vi "Barcode-Indentify-Sort(Include-Read)_Api.vi"(8 "Error In":errorcluster, 11 "Progressing Data":T5) -> (0 "Error Out":errorcluster, 1 "輸出顏色-位置":T1(array[cluster]), 2 "Image":T2(plugin-control), 3 "Progressing Data":T5, 4 "第一次輸出結果(含排序)":cluster{"X值":dbl, "Data":string}[](array[cluster]), 5 "Barcodes":T3(array[cluster]) {"Confidence Level" format="%.2f"; "Barcode Type" items=["Reserved", "Codabar", "Code 39", "Code 93", "Code 128", "EAN 8", "EAN 13", "Interleaved 2 of 5", "MSI", "UPCA", "Pharmacode", "RSS Limited"]; "Bounding Box"."y" format="%.2f"; "Bounding Box"."x" format="%.2f"})   [LabVIEW 2019]
uses:
  <vilib>/vision/Image Controls.llb/IMAQ Image.ctl
  <vilib>/userDefined/High Color/IMAQdx.ctl
  <vilib>/myRIO/Instrument Drivers/Onboard IO/DIO/typedefs/DIO Reference.ctl
  <vilib>/myRIO/Common/Instrument Driver Framework/Utilities/typedefs/myRIO Generic Hardware Reference.ctl
  <vilib>/myRIO/Common/Instrument Driver Framework/Utilities/typedefs/Hardware Version Enum.ctl
  <vilib>/myRIO/Common/Instrument Driver Framework/Utilities/typedefs/myRIO v1.0 Reference.ctl
  <vilib>/myRIO/Common/Instrument Driver Framework/Utilities/typedefs/Generic FPGA Reference.ctl
  <vilib>/myRIO/Common/Instrument Driver Framework/myRIO v1.0/DIO/typedefs/DIO Channels List.ctl
  <vilib>/myRIO/Common/Instrument Driver Framework/myRIO v1.0/DIO/typedefs/DIO Channels Enum.ctl
  <vilib>/userDefined/High Color/nirio_resource_hc.ctl
  <vilib>/myRIO/Common/Instrument Driver Framework/Utilities/vis/Is FPGA Ref Available.vi
  <vilib>/myRIO/Common/Instrument Driver Framework/myRIO v1.0/DIO/vis/myRIO v1.1 Open DIO.vi
  <vilib>/myRIO/Instrument Drivers/Onboard IO/DIO/vis/Write.vi
  <vilib>/myRIO/Common/Instrument Driver Framework/Utilities/vis/Validate Channels.vi
  <vilib>/myRIO/Common/Instrument Driver Framework/myRIO v1.0/DIO/vis/myRIO v1.0 Reserve DIO.vi
  <vilib>/myRIO/Common/Instrument Driver Framework/myRIO v1.0/Resource Manager/vis/myRIO v1.0 Reserve Channel List.vi
  <vilib>/myRIO/Common/Instrument Driver Framework/myRIO v1.0/DIO/vis/myRIO v1.0 Build MUX Configuration DIO.vi
  <vilib>/myRIO/Common/Instrument Driver Framework/myRIO v1.0/Resource Manager/vis/myRIO v1.0 Reserve Channel.vi
  <vilib>/myRIO/Common/Instrument Driver Framework/myRIO v1.0/Resource Manager/vis/myRIO v1.0 Unreserve Channel.vi
  <vilib>/myRIO/Common/Instrument Driver Framework/myRIO v1.0/Resource Manager/vis/myRIO v1.0 Create Configuration List.vi
  <vilib>/myRIO/Common/Instrument Driver Framework/myRIO v1.0/Resource Manager/vis/myRIO v1.0 Build Mutex Name.vi
  <vilib>/Utility/VariantDataType/GetNumericInfo.vi
  <vilib>/Utility/error.llb/Error Cluster From Error Code.vi
  <vilib>/myRIO/Common/Instrument Driver Framework/myRIO v1.0/myRIO v1.1 Open.vi
  <vilib>/myRIO/Common/Instrument Driver Framework/Utilities/vis/IO Manager.vi
  <vilib>/myRIO/Common/Instrument Driver Framework/Utilities/vis/Configuration Manager.vi
  <vilib>/myRIO/Common/Instrument Driver Framework/myRIO v1.0/Resource Manager/vis/myRIO v1.0 Configure IO.vi
  <vilib>/myRIO/Common/Instrument Driver Framework/myRIO v1.0/myRIO v1.0 Close.vi
  <vilib>/myRIO/Common/Instrument Driver Framework/myRIO v1.0/DIO/vis/myRIO v1.0 Write DIO.vi
  <vilib>/myRIO/Express VI/Onboard Devices/LED/LED Express VI.xnode
  <vilib>/myRIO/Instrument Drivers/Onboard IO/DIO/vis/myRIO DIO Open.xnode
  <vilib>/myRIO/Instrument Drivers/Onboard IO/DIO/DIO.lvlib
panel:
  out "第二次輸出結果(含排序)":cluster{"x":dbl, "Data":string}[](array[cluster])
  out "排完順序的辨識結果":cluster{"Numeric":dbl, "Data":string}[](array[cluster])
  in  "Stop 2":bool
  out "Image 2":T2(plugin-control)
  out "Barcodes 2":T3(array[cluster]) {"Confidence Level" format="%.2f"; "Barcode Type" items=["Reserved", "Codabar", "Code 39", "Code 93", "Code 128", "EAN 8", "EAN 13", "Interleaved 2 of 5", "MSI", "UPCA", "Pharmacode", "RSS Limited"]; "Bounding Box"."y" format="%.2f"; "Bounding Box"."x" format="%.2f"}
  in  "Stop":bool
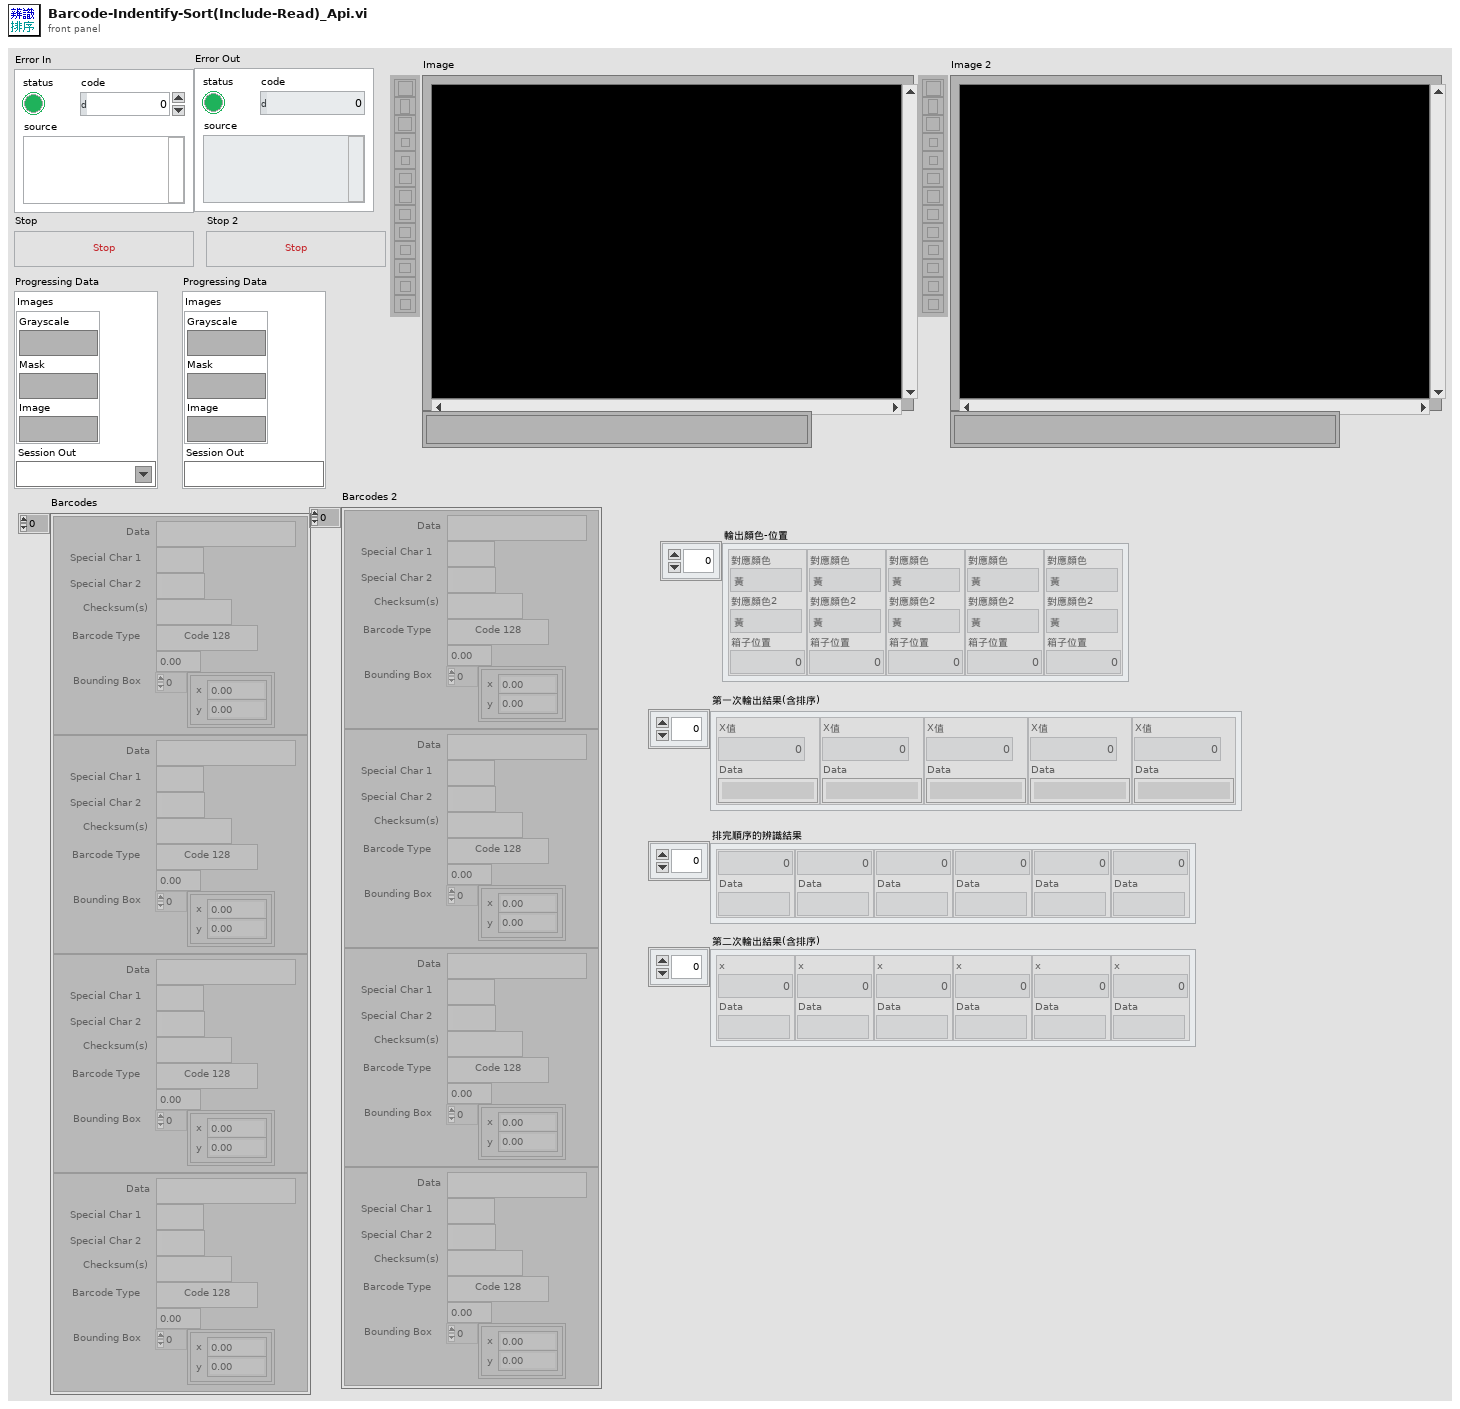
[diagram p1: front panel]
types:
  T1 = cluster{"對應顏色":enum16{"黃", "紅", "綠", "藍", "黑"}, "對應顏色2":enum16{"黃", "紅", "綠", "藍", "黑"}, "箱子位置":i32}[]
  T2 = typedef "IMAQ Image.ctl" = refnum<image>
  T3 = cluster{"Data":string, "Special Char 1":string, "Special Char 2":string, "Checksum(s)":string, "Barcode Type":u32, "Confidence Level":sgl, "Bounding Box":cluster{"x":sgl, "y":sgl}[]}[]
  T4 = typedef "IMAQdx.ctl" = refnum<k21>
  T5 = cluster{"Images":cluster{"Grayscale":T2, "Mask":T2, "Image":T2}, "Session Out":T4}
  T6 = typedef "DIO.lvlib/DIO Reference.ctl" = cluster{"myRIO Reference":T7, "DIO Channels List":T11}
  T7 = typedef "myRIO Generic Hardware Reference.ctl" = cluster{"myRIO Model":T8, "myRIO Hardware Reference":T9}
  T8 = typedef "Hardware Version Enum.ctl" = enum16{"Unknown", "myRIO-1900", "myRIO-1950", "roboRIO", "NI ELVIS RIO CM", "ELVIS III"}
  T9 = typedef "myRIO v1.0 Reference.ctl" = cluster{"Generic FPGA Reference":T10, "Allow multiple opens":bool}
  T10 = typedef "Generic FPGA Reference.ctl" = refnum<k20>
  T11 = typedef "DIO Channels List.ctl" = T12[]
  T12 = typedef "DIO Channels Enum.ctl" = enum16{"Not Connected", "C/DIO0", "C/DIO1", "C/DIO2", "C/DIO3", "C/DIO4", "C/DIO5", "C/DIO6", "C/DIO7", "A/DIO0", "A/DIO1", "A/DIO2", "A/DIO3", "A/DIO4", "A/DIO5", "A/DIO6", "A/DIO7", "A/DIO8", "A/DIO9", "A/DIO10", "A/DIO11", "A/DIO12", "A/DIO13", "A/DIO14", "A/DIO15", "A/DIO16", "A/DIO17", "A/DIO18", "A/DIO19", "B/DIO0", "B/DIO1", "B/DIO2", "B/DIO3", "B/DIO4", "B/DIO5", "B/DIO6", "B/DIO7", "B/DIO8", "B/DIO9", "B/DIO10", "B/DIO11", "B/DIO12", "B/DIO13", "B/DIO14", "B/DIO15", "B/DIO16", "B/DIO17", "B/DIO18", "B/DIO19", "LED0", "LED1", "LED2", "LED3", "Button0", "DIO/DIO0", "DIO/DIO1", "DIO/DIO2", "DIO/DIO3", "DIO/DIO4", "DIO/DIO5", "DIO/DIO6", "DIO/DIO7", "DIO/DIO8", "DIO/DIO9", "SPI/CS0", "SPI/CS1", "SPI/CS2", "SPI/CS3", "LED RADIO (Green)", "LED RADIO (Red)", "LED COMM (Green)", "LED COMM (Red)", "LED MODE (Green)", "LED MODE (Red)"}
  T13 = typedef "nirio_resource_hc.ctl" = tag
  T14 = cluster{"對應顏色":enum16{"黃", "紅", "綠", "藍", "黑"}, "對應顏色2":enum16{"黃", "紅", "綠", "藍", "黑"}, "箱子位置":i32}
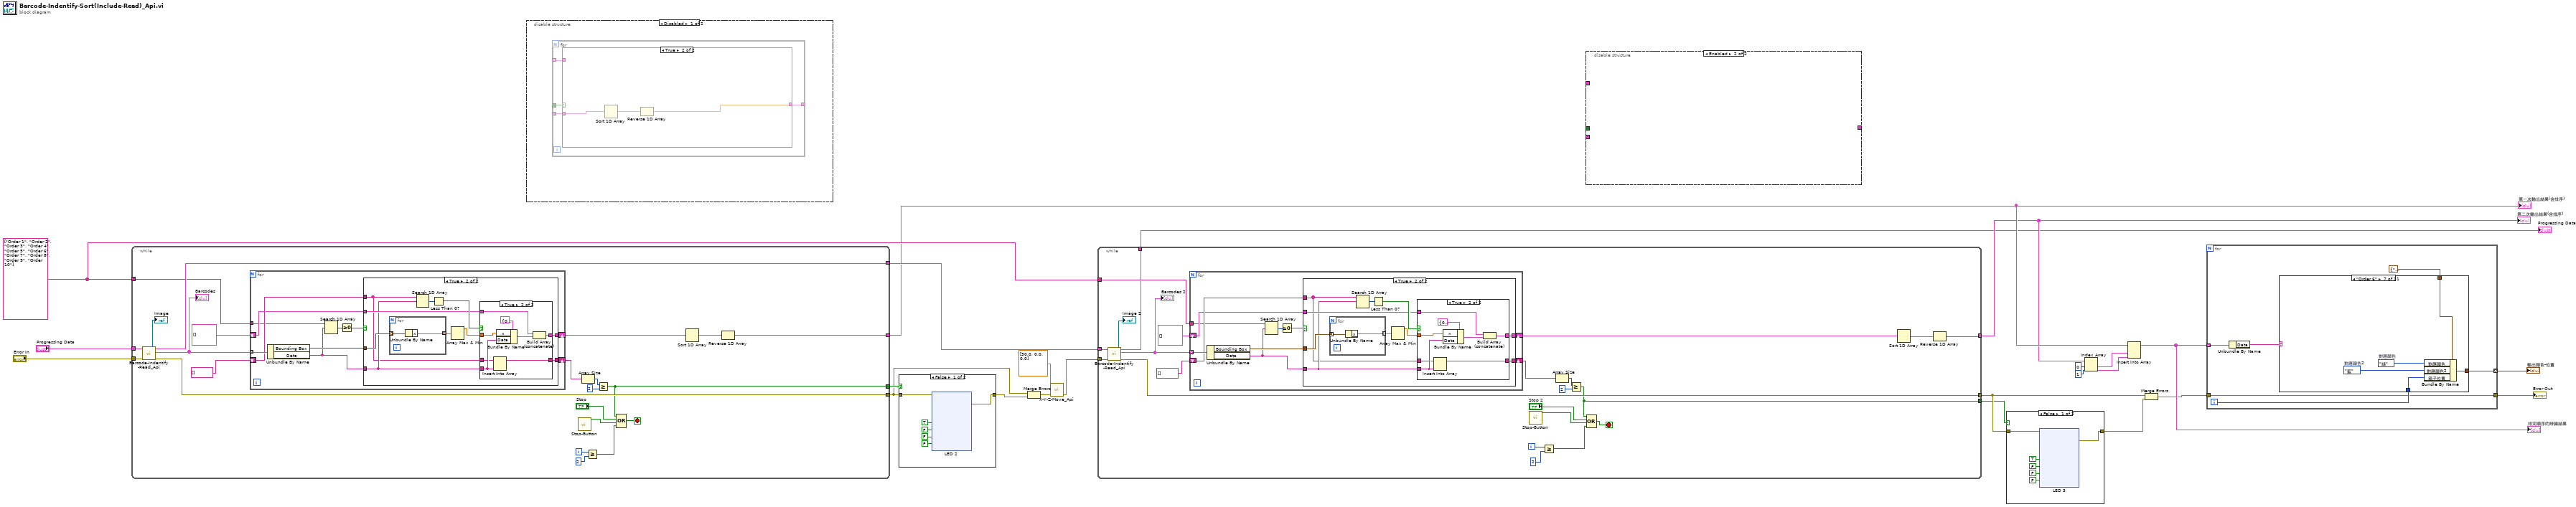
[diagram p0: block diagram]
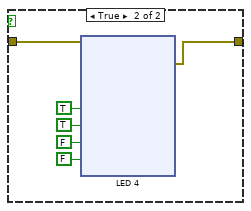
[diagram p2: hidden frame]
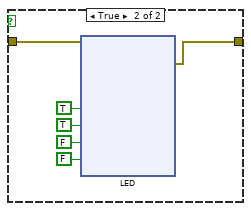
[diagram p3: hidden frame]
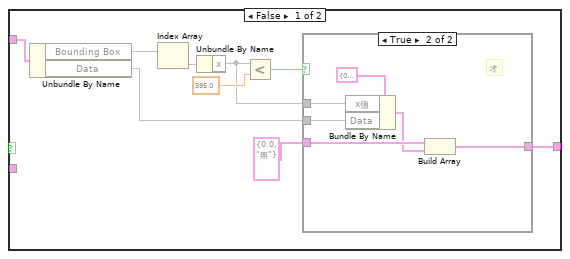
[diagram p4: hidden frame]
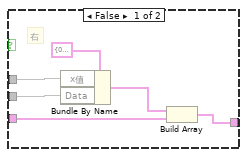
[diagram p5: hidden frame]
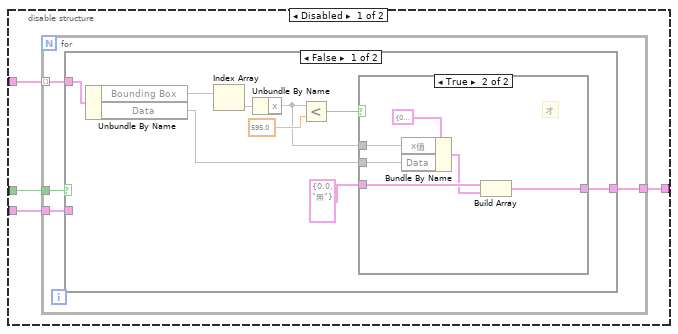
[diagram p7: hidden frame]
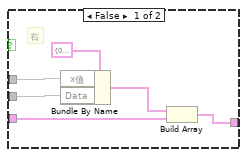
[diagram p8: hidden frame]
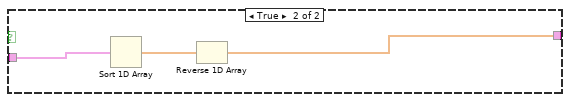
[diagram p9: hidden frame]
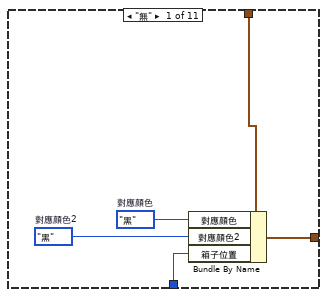
[diagram p10: hidden frame]
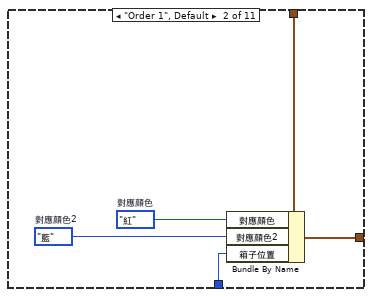
[diagram p11: hidden frame]
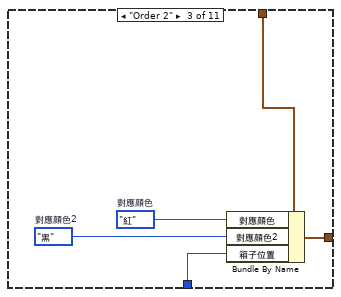
[diagram p12: hidden frame]
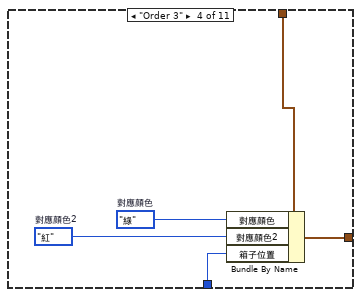
[diagram p13: hidden frame]
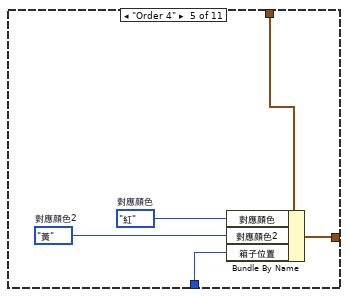
[diagram p14: hidden frame]
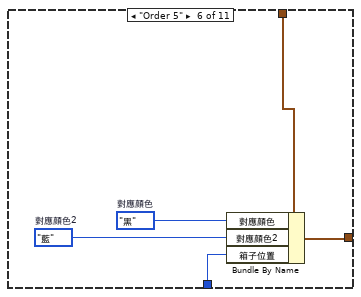
[diagram p15: hidden frame]
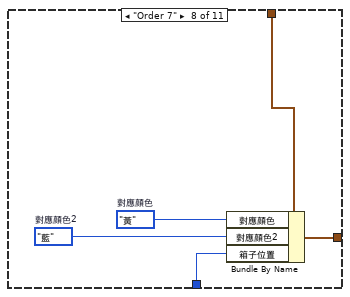
[diagram p16: hidden frame]
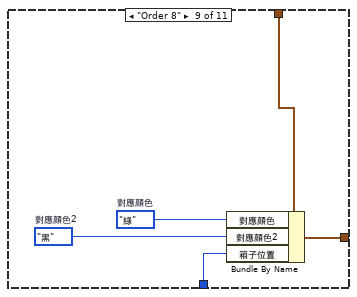
[diagram p17: hidden frame]
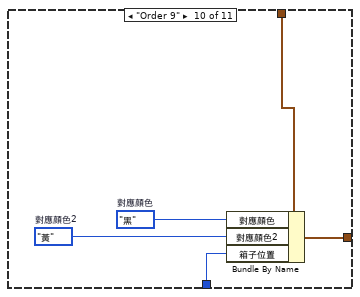
[diagram p18: hidden frame]
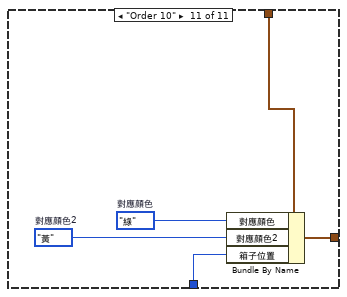
[diagram p19: hidden frame]
diagram:
  w21 = string[] ["Order 1", "Order 2", "Order 3", "Order 4", "Order 5", "Order 6", "Order 7", "Order 8", "Order 9", "Order 10"]
  n1 = while {
    tunnel: "Error In" -> [w33]
    tunnel: [w26] -> w14
    tunnel: [w34] -> w5
    tunnel: "Progressing Data" -> [w40]
    tunnel: [w39] -> w22
    tunnel: w21 -> [w36]
    tunnel: [w25] -> w8
    i -> [w32]
    stop <- w42 stop-if-true
    n2 = call "Barcode-Indentify-Read_Api.vi"("Error In"=w33, "Progressing Data"=w40) -> ("Error Out"=w34:errorcluster, "Barcodes"=w29:T3, "Progressing Data"=w39:T5, "Image"=→"Image":T2)  [unwired: 6 in]
    "Barcodes" <- w29
    n3 = for {
      tunnel: w29 -> [w56] mode=indexing
      shift-right: [w51] -> w35
      shift-left: string[] [] -> [w53]
      shift-right: [w54] -> w27
      shift-left: cluster{sgl, "Data":string}[] [] -> [w52]
      tunnel: w36 -> [w48]
      n4 = Unbundle By Name(w56) -> ("Bounding Box"=w55:cluster{"x":sgl, "y":sgl}[], "Data"=w47:string)
      n5 = Search 1D Array(1D array=w48, element=w47) -> (index of element=w50:i32)  [unwired: 1 in]
      n6 = Greater Or Equal To 0?(x=w50) -> (x >= 0?=w49:bool)
      n7 = case shown="True" w49 {
        tunnel: w55 -> [_ w68]
        tunnel: [w57 w66] -> w54
        tunnel: w47 -> [_ w61]
        tunnel: w53 -> [w58 w60]
        tunnel: w52 -> [w57 w63]
        tunnel: [w58 w62] -> w51
        frame False {
        }
        frame True {
          n8 = for {
            tunnel: w68 -> [w80] mode=indexing
            tunnel: [w79] -> w67 mode=indexing
            n9 = Unbundle By Name(w80) -> ("x"=w79:sgl)
          }
          n10 = Search 1D Array(1D array=w60, element=w61) -> (index of element=w65:i32)  [unwired: 1 in]
          n11 = Less Than 0?(x=w65) -> (x < 0?=w64:bool)
          n12 = Array Max & Min(array=w67) -> (max value=w59:sgl)  [unwired: 3 out]
          n13 = case shown="True" w64 {
            tunnel: w59 -> [_ w78]
            tunnel: w61 -> [_ w76]
            tunnel: [w69 w77] -> w66
            tunnel: w60 -> [w70 w75]
            tunnel: [w70 w74] -> w62
            tunnel: w63 -> [w69 w73]
            frame False {
            }
            frame True {
              n14 = Insert Into Array "Insert Into Array"(array=w75, new element=w76) -> (w74:string[])  [unwired: 1 in]
              n15 = Bundle By Name(cluster=cluster{"x":dbl, "Data":string} {"x"=0.0, "Data"=""} ("input cluster"), "x"=w78, "Data"=w76) -> (w72:cluster{"x":dbl, "Data":string})
              n16 = Build Array (concatenate)(w73, w72) -> (w77:cluster{"x":dbl, "Data":string}[])
            }
          }
        }
      }
    }
    n17 = call "Stop-Button.vi"() -> ("顯示按下?"=w38:bool)  [unwired: 10 in, 1 out]
    n18 = Array Size(array=w35) -> (size(s)=w44:i32)
    n19 = Greater Or Equal?(x=w32, y=2) -> (x >= y?=w31:bool)
    n20 = Greater Or Equal?(x=w44, y=2) -> (x >= y?=w25:bool)
    n21 = Compound Arithmetic op=OR(w25, "Stop", w38, w31) -> (w42:bool)
    n22 = Sort 1D Array(array=w27) -> (sorted array=w28:cluster{"x":dbl, "Data":string}[])
    n23 = Reverse 1D Array(array=w28) -> (reversed array=w26:cluster{"x":dbl, "Data":string}[])
  }
  "第一次輸出結果(含排序)" <- w14
  n24 = disable-structure shown="Disabled" {
    frame Disabled {
      n25 = for {
        tunnel: [w84] -> _
        tunnel: _ -> [w83]
        tunnel: _ -> [w82]
        tunnel: _ -> [w81] mode=indexing
        n26 = case shown="True" w82 {
          tunnel: [w85 w108] -> w84
          tunnel: w83 -> [_ w106]
          tunnel: w81 -> [w89 _]
          frame False {
            n27 = Unbundle By Name(w89) -> ("Bounding Box"=w93, "Data"=w88)
            n28 = Index Array(array=w93) -> (element=w92)  [unwired: 1 in]
            n29 = Unbundle By Name(w92) -> ("x"=w87)
            n30 = Less?(x=w87, y=sgl 595.0) -> (x < y?=w90:bool)
            n31 = case shown="True" w90 {
              tunnel: w88 -> [w98 w105]
              tunnel: w87 -> [w97 w104]
              tunnel: cluster{"x值":dbl, "Data":string} {"x值"=0.0, "Data"="無"} ("element") -> [w95 w101]
              tunnel: [w96 w102] -> w85
              frame False {
                # "右"
                n32 = Bundle By Name(cluster=cluster{"x值":dbl, "Data":string} {"x值"=0.0, "Data"=""} ("input cluster"), "x值"=w97, "Data"=w98) -> (w94:cluster{"x值":dbl, "Data":string})
                n33 = Build Array(w94, w95) -> (w96:cluster{"x值":dbl, "Data":string}[])
              }
              frame True {
                # "オ"
                n34 = Bundle By Name(cluster=cluster{"x值":dbl, "Data":string} {"x值"=0.0, "Data"=""} ("input cluster"), "x值"=w104, "Data"=w105) -> (w100:cluster{"x值":dbl, "Data":string})
                n35 = Build Array(w101, w100) -> (w102:cluster{"x值":dbl, "Data":string}[])
              }
            }
          }
          frame True {
            n36 = Sort 1D Array(array=w106) -> (sorted array=w107:ext[])
            n37 = Reverse 1D Array(array=w107) -> (reversed array=w108:ext[])
          }
        }
      }
    }
    frame Enabled {
    }
  }
  n38 = case shown="False" w8 {
    tunnel: w5 -> [w109 w158]
    tunnel: [w110 w153] -> w6
    frame False {
      n39 = xnode "LED 2"("LED0"=TRUE, "LED1"=FALSE, "LED2"=FALSE, "LED3"=FALSE, "error in (no error)"=w109) -> ("error out"=w110:errorcluster)
    }
    frame True {
      n40 = xnode "LED"("LED0"=TRUE, "LED1"=TRUE, "LED2"=FALSE, "LED3"=FALSE, "error in (no error)"=w158) -> ("error out"=w153:errorcluster)
    }
  }
  n41 = Merge Errors(w5, w6) -> (w7:errorcluster)
  n42 = call "X-Y-Z-Move_Api.vi"("Error In"=w7, "X-Y-Z移動"=dbl[] [50.0, 0.0, 0.0]) -> ("Error Out"=w23:errorcluster)  [unwired: 8 in, 1 out]
  n43 = while {
    tunnel: w23 -> [w217]
    tunnel: [w199] -> w13
    tunnel: [w206] -> w3
    tunnel: w22 -> [w211]
    tunnel: w21 -> [w208]
    tunnel: [w201] -> w9
    tunnel: [w197] -> w1
    i -> [w204]
    stop <- w213 stop-if-true
    n44 = call "Barcode-Indentify-Read_Api.vi"("Error In"=w217, "Progressing Data"=w211) -> ("Error Out"=w206:errorcluster, "Barcodes"=w202:T3, "Progressing Data"=w201:T5, "Image"=→"Image 2":T2)  [unwired: 6 in]
    "Barcodes 2" <- w202
    n45 = for {
      tunnel: w202 -> [w228] mode=indexing
      shift-right: [w223] -> w207
      shift-left: string[] [] -> [w225]
      shift-right: [w226] -> w198
      shift-left: cluster{sgl, "Data":string}[] [] -> [w224]
      tunnel: w208 -> [w220]
      n46 = Unbundle By Name(w228) -> ("Bounding Box"=w227:cluster{"x":sgl, "y":sgl}[], "Data"=w219:string)
      n47 = Search 1D Array(1D array=w220, element=w219) -> (index of element=w222:i32)  [unwired: 1 in]
      n48 = Greater Or Equal To 0?(x=w222) -> (x >= 0?=w221:bool)
      n49 = case shown="True" w221 {
        tunnel: w227 -> [_ w240]
        tunnel: [w229 w238] -> w226
        tunnel: w219 -> [_ w233]
        tunnel: w225 -> [w230 w232]
        tunnel: w224 -> [w229 w235]
        tunnel: [w230 w234] -> w223
        frame False {
        }
        frame True {
          n50 = for {
            tunnel: w240 -> [w252] mode=indexing
            tunnel: [w251] -> w239 mode=indexing
            n51 = Unbundle By Name(w252) -> ("x"=w251:sgl)
          }
          n52 = Search 1D Array(1D array=w232, element=w233) -> (index of element=w237:i32)  [unwired: 1 in]
          n53 = Less Than 0?(x=w237) -> (x < 0?=w236:bool)
          n54 = Array Max & Min(array=w239) -> (max value=w231:sgl)  [unwired: 3 out]
          n55 = case shown="True" w236 {
            tunnel: w231 -> [_ w250]
            tunnel: w233 -> [_ w248]
            tunnel: [w241 w249] -> w238
            tunnel: w232 -> [w242 w247]
            tunnel: [w242 w246] -> w234
            tunnel: w235 -> [w241 w245]
            frame False {
            }
            frame True {
              n56 = Insert Into Array "Insert Into Array"(array=w247, new element=w248) -> (w246:string[])  [unwired: 1 in]
              n57 = Bundle By Name(cluster=cluster{"x":dbl, "Data":string} {"x"=0.0, "Data"=""} ("input cluster"), "x"=w250, "Data"=w248) -> (w244:cluster{"x":dbl, "Data":string})
              n58 = Build Array (concatenate)(w245, w244) -> (w249:cluster{"x":dbl, "Data":string}[])
            }
          }
        }
      }
    }
    n59 = call "Stop-Button.vi"() -> ("顯示按下?"=w210:bool)  [unwired: 10 in, 1 out]
    n60 = Greater Or Equal?(x=w204, y=2) -> (x >= y?=w205:bool)
    n61 = Array Size(array=w207) -> (size(s)=w215:i32)
    n62 = Greater Or Equal?(x=w215, y=2) -> (x >= y?=w197:bool)
    n63 = Compound Arithmetic op=OR(w197, "Stop 2", w210, w205) -> (w213:bool)
    n64 = Sort 1D Array(array=w198) -> (sorted array=w200:cluster{"x":dbl, "Data":string}[])
    n65 = Reverse 1D Array(array=w200) -> (reversed array=w199:cluster{"x":dbl, "Data":string}[])
  }
  "Progressing Data" <- w9
  "第二次輸出結果(含排序)" <- w13
  n66 = disable-structure shown="Enabled" {
    disable-tunnel: _ -> [w256 _]
    disable-tunnel: _ -> [w255 _]
    disable-tunnel: _ -> [w254 _]
    disable-tunnel: [w253 _] -> _
    frame Disabled {
      n67 = for {
        tunnel: [w260] -> w253
        tunnel: w255 -> [w259]
        tunnel: w256 -> [w258]
        tunnel: w254 -> [w257] mode=indexing
        n68 = case shown="False" w258 {
          tunnel: [w261 w284] -> w260
          tunnel: w259 -> [_ w282]
          tunnel: w257 -> [w265 _]
          frame False {
            n69 = Unbundle By Name(w265) -> ("Bounding Box"=w269, "Data"=w264)
            n70 = Index Array(array=w269) -> (element=w268)  [unwired: 1 in]
            n71 = Unbundle By Name(w268) -> ("x"=w263)
            n72 = Less?(x=w263, y=sgl 595.0) -> (x < y?=w266:bool)
            n73 = case shown="True" w266 {
              tunnel: w264 -> [w274 w281]
              tunnel: w263 -> [w273 w280]
              tunnel: cluster{"x值":dbl, "Data":string} {"x值"=0.0, "Data"="無"} ("element") -> [w271 w277]
              tunnel: [w272 w278] -> w261
              frame False {
                # "右"
                n74 = Bundle By Name(cluster=cluster{"x值":dbl, "Data":string} {"x值"=0.0, "Data"=""} ("input cluster"), "x值"=w273, "Data"=w274) -> (w270:cluster{"x值":dbl, "Data":string})
                n75 = Build Array(w270, w271) -> (w272:cluster{"x值":dbl, "Data":string}[])
              }
              frame True {
                # "オ"
                n76 = Bundle By Name(cluster=cluster{"x值":dbl, "Data":string} {"x值"=0.0, "Data"=""} ("input cluster"), "x值"=w280, "Data"=w281) -> (w276:cluster{"x值":dbl, "Data":string})
                n77 = Build Array(w277, w276) -> (w278:cluster{"x值":dbl, "Data":string}[])
              }
            }
          }
          frame True {
            n78 = Sort 1D Array(array=w282) -> (sorted array=w283:ext[])
            n79 = Reverse 1D Array(array=w283) -> (reversed array=w284:ext[])
          }
        }
      }
    }
    frame Enabled {
    }
  }
  n80 = case shown="False" w1 {
    tunnel: w3 -> [w285 w334]
    tunnel: [w286 w329] -> w2
    frame False {
      n81 = xnode "LED 3"("LED0"=TRUE, "LED1"=FALSE, "LED2"=FALSE, "LED3"=FALSE, "error in (no error)"=w285) -> ("error out"=w286:errorcluster)
    }
    frame True {
      n82 = xnode "LED 4"("LED0"=TRUE, "LED1"=TRUE, "LED2"=FALSE, "LED3"=FALSE, "error in (no error)"=w334) -> ("error out"=w329:errorcluster)
    }
  }
  n83 = Index Array(array=w13, index #1=0 ("index"), index #2=1 ("index")) -> (element #1=w16:cluster{"x":dbl, "Data":string}, element #2=w15:cluster{"x":dbl, "Data":string})
  n84 = Insert Into Array(array=w14, new element #1=w16, new element #2=w15) -> (w12:cluster{"x":dbl, "Data":string}[])  [unwired: 1 in]
  "排完順序的辨識結果" <- w12
  n85 = Merge Errors(w3, w2) -> (w4:errorcluster)
  n86 = for {
    tunnel: [w377] -> w11 mode=indexing
    tunnel: w12 -> [w376] mode=indexing
    tunnel: [w374] -> w10
    tunnel: w4 -> [w374]
    i -> [w378]
    n87 = Unbundle By Name(w376) -> ("Data"=w375:string)
    n88 = case shown="\"Order 6\"" w375 {
      tunnel: w378 -> [w382 w388 w390 w396 w400 w405 w410 w415 w420 w425 w430]
      tunnel: [w383 w387 w391 w395 w401 w406 w411 w416 w421 w426 w431] -> w377
      tunnel: T14 {"對應顏色"=enum."黃", "對應顏色2"=enum."黃", "箱子位置"=0} ("input cluster") -> [w381 w384 w389 w394 w399 w404 w409 w414 w419 w424 w429]
      frame "無" {
        w379 = enum16{"黃", "紅", "綠", "藍", "黑"}."黑"  # 對應顏色2
        w380 = enum16{"黃", "紅", "綠", "藍", "黑"}."黑"  # 對應顏色
        n89 = Bundle By Name(cluster=w381, "對應顏色"=w380, "對應顏色2"=w379, "箱子位置"=w382) -> (w383:T14)
      }
      frame "Order 1", Default {
        w385 = enum16{"黃", "紅", "綠", "藍", "黑"}."藍"  # 對應顏色2
        w386 = enum16{"黃", "紅", "綠", "藍", "黑"}."紅"  # 對應顏色
        n90 = Bundle By Name(cluster=w384, "對應顏色"=w386, "對應顏色2"=w385, "箱子位置"=w388) -> (w387:T14)
      }
      frame "Order 2" {
        w392 = enum16{"黃", "紅", "綠", "藍", "黑"}."黑"  # 對應顏色2
        w393 = enum16{"黃", "紅", "綠", "藍", "黑"}."紅"  # 對應顏色
        n91 = Bundle By Name(cluster=w389, "對應顏色"=w393, "對應顏色2"=w392, "箱子位置"=w390) -> (w391:T14)
      }
      frame "Order 3" {
        w397 = enum16{"黃", "紅", "綠", "藍", "黑"}."紅"  # 對應顏色2
        w398 = enum16{"黃", "紅", "綠", "藍", "黑"}."綠"  # 對應顏色
        n92 = Bundle By Name(cluster=w394, "對應顏色"=w398, "對應顏色2"=w397, "箱子位置"=w396) -> (w395:T14)
      }
      frame "Order 4" {
        w402 = enum16{"黃", "紅", "綠", "藍", "黑"}."黃"  # 對應顏色2
        w403 = enum16{"黃", "紅", "綠", "藍", "黑"}."紅"  # 對應顏色
        n93 = Bundle By Name(cluster=w399, "對應顏色"=w403, "對應顏色2"=w402, "箱子位置"=w400) -> (w401:T14)
      }
      frame "Order 5" {
        w407 = enum16{"黃", "紅", "綠", "藍", "黑"}."藍"  # 對應顏色2
        w408 = enum16{"黃", "紅", "綠", "藍", "黑"}."黑"  # 對應顏色
        n94 = Bundle By Name(cluster=w404, "對應顏色"=w408, "對應顏色2"=w407, "箱子位置"=w405) -> (w406:T14)
      }
      frame "Order 6" {
        w412 = enum16{"黃", "紅", "綠", "藍", "黑"}."藍"  # 對應顏色2
        w413 = enum16{"黃", "紅", "綠", "藍", "黑"}."綠"  # 對應顏色
        n95 = Bundle By Name(cluster=w409, "對應顏色"=w413, "對應顏色2"=w412, "箱子位置"=w410) -> (w411:T14)
      }
      frame "Order 7" {
        w417 = enum16{"黃", "紅", "綠", "藍", "黑"}."藍"  # 對應顏色2
        w418 = enum16{"黃", "紅", "綠", "藍", "黑"}."黃"  # 對應顏色
        n96 = Bundle By Name(cluster=w414, "對應顏色"=w418, "對應顏色2"=w417, "箱子位置"=w415) -> (w416:T14)
      }
      frame "Order 8" {
        w422 = enum16{"黃", "紅", "綠", "藍", "黑"}."黑"  # 對應顏色2
        w423 = enum16{"黃", "紅", "綠", "藍", "黑"}."綠"  # 對應顏色
        n97 = Bundle By Name(cluster=w419, "對應顏色"=w423, "對應顏色2"=w422, "箱子位置"=w420) -> (w421:T14)
      }
      frame "Order 9" {
        w427 = enum16{"黃", "紅", "綠", "藍", "黑"}."黃"  # 對應顏色2
        w428 = enum16{"黃", "紅", "綠", "藍", "黑"}."黑"  # 對應顏色
        n98 = Bundle By Name(cluster=w424, "對應顏色"=w428, "對應顏色2"=w427, "箱子位置"=w425) -> (w426:T14)
      }
      frame "Order 10" {
        w432 = enum16{"黃", "紅", "綠", "藍", "黑"}."黃"  # 對應顏色2
        w433 = enum16{"黃", "紅", "綠", "藍", "黑"}."綠"  # 對應顏色
        n99 = Bundle By Name(cluster=w429, "對應顏色"=w433, "對應顏色2"=w432, "箱子位置"=w430) -> (w431:T14)
      }
    }
  }
  "Error Out" <- w10
  "輸出顏色-位置" <- w11
